vi "mltcoreimaqdx_final.vi"() -> ()   [LabVIEW 2014]
doc: "The Grab VI acquires images continuously and displays the images in an image control using low-level acquisition VIs. A grab is appropriate for high-speed applications in which you need to process only one image at a time."
uses:
  <vilib>/userdefined/High Color/IMAQdx.ctl
  <vilib>/vision/driver/IMAQdx.llb/IMAQdx Acquisition Mode.ctl
  <vilib>/vision/driver/IMAQdx.llb/IMAQdx Buffer Number Mode.ctl
  <vilib>/vision/driver/NI_Vision_Acquisition_Software.lvlib
  <vilib>/vision/NI_Vision_Development_Module.lvlib
panel:
  in  "Add Delay to process loop (ms)":u32
  out "# elements in queue":i32(knob) scale=0.0..250.0
  in  "Range":cluster{"Lower value":sgl, "Upper value":sgl}={"Lower value"=50.0, "Upper value"=140.0} {"Upper value" format="%.2f"; "Lower value" format="%.2f"}
  out "Acquired Image":T1(plugin-control)
  out "Processed Image":T1(plugin-control)
  in  "IMAQdx Session":T2="cam0"
  out "ProcessFrameRate":dbl(knob) scale=0.0..100.0 scale format="%.1f"
  out "ProcessBufferNumber":u32
  out "CameraBuffer Number":u32
  out "CameraFrameRate":dbl(knob) scale=0.0..100.0 scale format="%.1f"
  in  "stop":bool
  # "This example uses NI-IMAQdx to acquire images\nand utilizes a Producer/Consumer loop architecture\nto split the image acquisition and image processing\nbetween multiple threads."
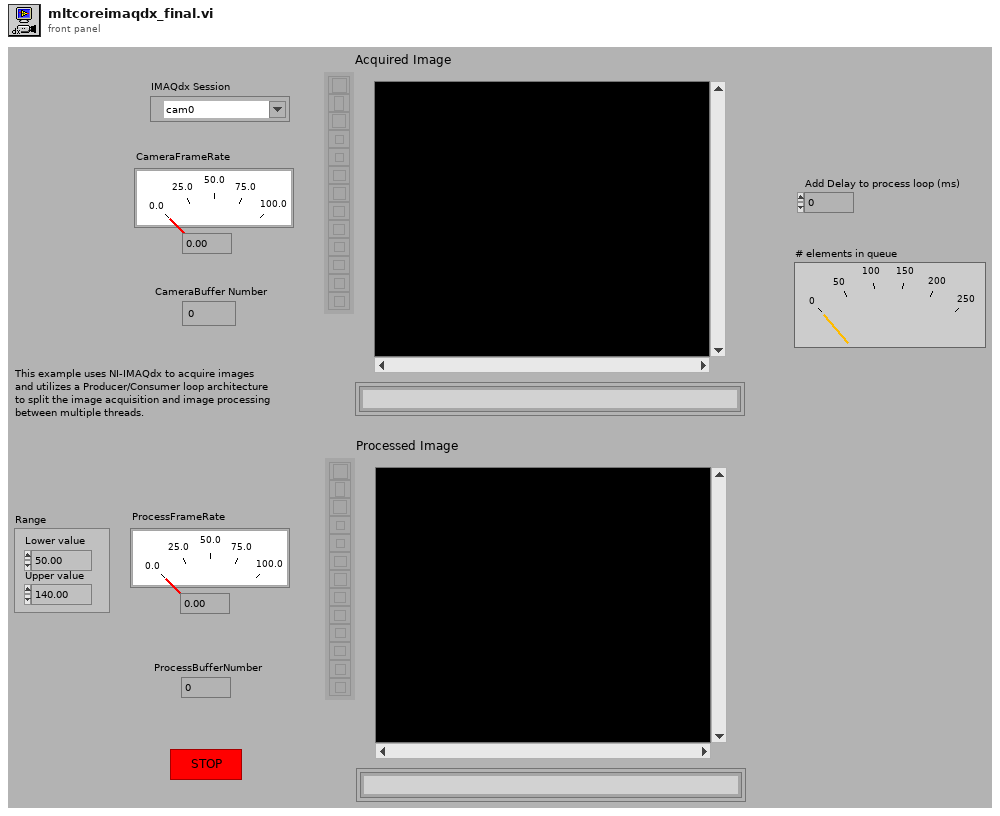
[diagram p1: front panel]
types:
  T1 = typedef "IMAQ Image.ctl" = refnum<image>
  T2 = typedef "IMAQdx.ctl" = refnum<k21>
  T3 = typedef "Image Type" = u32
  T4 = typedef "NI_Vision_Acquisition_Software.lvlib/IMAQdx Acquisition Mode.ctl" = enum32{"One Shot", "Continuous"}
  T5 = typedef "NI_Vision_Acquisition_Software.lvlib/IMAQdx Buffer Number Mode.ctl" = enum32{"Next", "Last", "Buffer Number"}
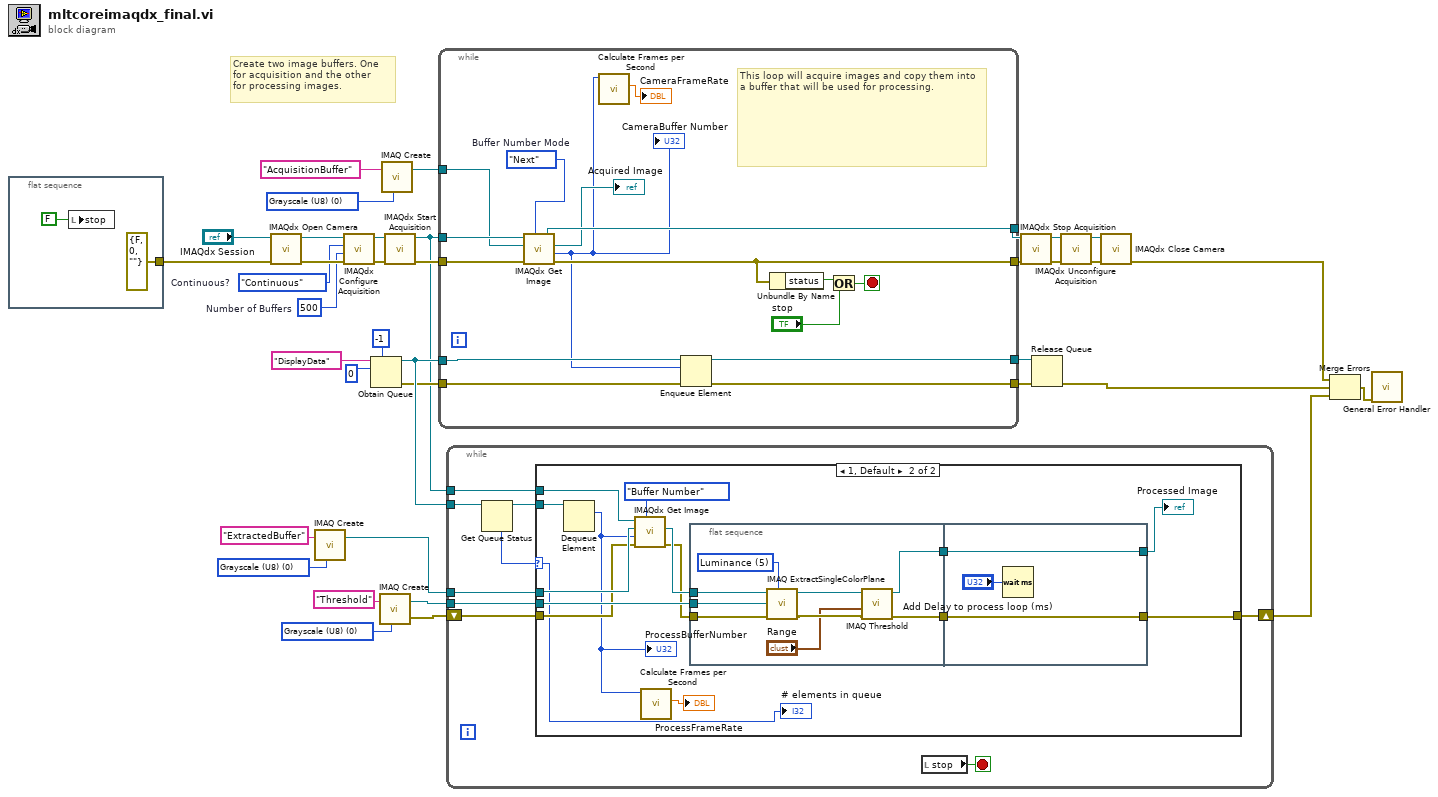
[diagram p0: block diagram]
diagram:
  w4 = T3 0 items=["Grayscale (U8)", "Grayscale (I16)", "Grayscale (SGL)", "Complex (CSG)", "RGB (U32)", "HSL (U32)", "RGB (U64)"] ("Image Type")
  w6 = T3 0 items=["Grayscale (U8)", "Grayscale (I16)", "Grayscale (SGL)", "Complex (CSG)", "RGB (U32)", "HSL (U32)", "RGB (U64)"] ("Image Type")
  w20 = T3 0 items=["Grayscale (U8)", "Grayscale (I16)", "Grayscale (SGL)", "Complex (CSG)", "RGB (U32)", "HSL (U32)", "RGB (U64)"] ("Image Type")
  w34 = u32 500  # Number of Buffers
  w12 = IMAQdx_Acquisition_Mode."Continuous"  # Continuous?
  # "Create two image buffers. One\nfor acquisition and the other\nfor processing images."
  n1 = flat-sequence {
    tunnel: [errorcluster {"status"=FALSE, "code"=0, "source"=""} ("error in")] -> w5
    frame #0 {
      n2 = local write "stop"(FALSE ("stop")) -> ()
    }
  }
  n3 = call <vilib>:"IMAQdx Open Camera.vi"("error in"=w5, "Session In"="IMAQdx Session") -> ("error out"=w35:errorcluster, "Session Out"=w36:T2)  [unwired: 8 in]
  n4 = call "IMAQ Create"("Image Name"="ExtractedBuffer", "Image Type"=w4) -> ("New Image"=w2:T1)  [unwired: 3 in, 1 out]
  n5 = call <vilib>:"IMAQdx Configure Acquisition.vi"("error in"=w35, "Number of Buffers"=w34, "Continuous?"=w12, "Session In"=w36) -> ("error out"=w15:errorcluster, "Session Out"=w11:T2)  [unwired: 6 in]
  n6 = Obtain Queue(max queue size (-1, unlimited)=-1, name (unnamed)="DisplayData", element data type=u32 0) -> (queue out=w23:refnum<queue>, error out=w21:errorcluster)  [unwired: 2 in, 1 out]
  n7 = call "IMAQ Create"("Image Name"="Threshold", "Image Type"=w6) -> ("New Image"=w8:T1, "error out"=w9:errorcluster)  [unwired: 3 in]
  n8 = call "IMAQ Create"("Image Name"="AcquisitionBuffer", "Image Type"=w20) -> ("New Image"=w37:T1)  [unwired: 3 in, 1 out]
  n9 = call <vilib>:"IMAQdx Start Acquisition.vi"("error in"=w15, "Session In"=w11) -> ("error out"=w14:errorcluster, "Session Out"=w1:T2)  [unwired: 8 in]
  n10 = while {
    tunnel: w14 -> [w51]
    tunnel: w1 -> [w52]
    tunnel: [w42] -> w33
    tunnel: w37 -> [w50]
    tunnel: [w49] -> w28
    tunnel: w23 -> [w48]
    tunnel: [w47] -> w24
    tunnel: [w46] -> w22
    tunnel: w21 -> [w45]
    stop <- w55 stop-if-true
    w44 = IMAQdx_Buffer_Number_Mode."Next"  # Buffer Number Mode
    # "This loop will acquire images and copy them into a buffer that will be used for processing."
    n11 = call <vilib>:"IMAQdx Get Image.vi"("Buffer Number Mode (Next)"=w44, "error in"=w51, "Image In"=w50, "Session In"=w52) -> ("error out"=w42:errorcluster, "Buffer Number Out"=w40:u32, "Image Out"=→"Acquired Image":T1, "Session Out"=w49:T2)  [unwired: 4 in]
    "CameraBuffer Number" <- w40
    n12 = call <vilib>:"Calculate Frames per Second.vi"("Buffer Number"=w40) -> ("Processed Frames/s"=→"CameraFrameRate":dbl)  [unwired: 8 in, 2 out]
    n13 = Enqueue Element(queue=w48, element=w40, error in (no error)=w45) -> (queue out=w47:refnum<queue>, error out=w46:errorcluster)  [unwired: 1 in, 1 out]
    n14 = Unbundle By Name(w42) -> ("status"=w54:bool)
    n15 = Or(x=w54, y="stop") -> (x .or. y?=w55:bool)
  }
  n16 = while {
    tunnel: w23 -> [w63]
    tunnel: w2 -> [w60]
    tunnel: w8 -> [w58]
    shift-right: [w57] -> w7
    shift-left: w9 -> [w59]
    tunnel: w1 -> [w56]
    stop <- w64 stop-if-true
    n17 = Get Queue Status(queue=w63) -> (queue out=w61:refnum<queue>, # elements in queue=w62:i32)  [unwired: 2 in, 6 out]
    n18 = case shown="1, Default" w62 {
      selector: w62 -> [_ w70]
      tunnel: w61 -> [_ w80]
      tunnel: w60 -> [_ w74]
      tunnel: w59 -> [w65 w72]
      tunnel: w58 -> [_ w79]
      tunnel: [w65 w78] -> w57
      tunnel: w56 -> [_ w76]
      frame 0 {
      }
      frame 1, Default {
        n19 = Dequeue Element(queue=w80) -> (element=w67:u32)  [unwired: 2 in, 3 out]
        "ProcessBufferNumber" <- w67
        n20 = call <vilib>:"IMAQdx Get Image.vi"("Buffer Number Mode (Next)"=IMAQdx_Buffer_Number_Mode."Buffer Number", "error in"=w72, "Buffer Number In"=w67, "Image In"=w74, "Session In"=w76) -> ("error out"=w71:errorcluster, "Image Out"=w73:T1)  [unwired: 3 in, 2 out]
        n21 = call <vilib>:"Calculate Frames per Second.vi"("Buffer Number"=w67) -> ("Processed Frames/s"=→"ProcessFrameRate":dbl)  [unwired: 8 in, 2 out]
        n22 = flat-sequence {
          tunnel: w79 -> [w89]
          tunnel: w73 -> [w82]
          tunnel: w71 -> [w81]
          tunnel: [w86] -> w69
          tunnel: [w84] -> w68
          tunnel: [w91] -> w77
          tunnel: [w92] -> w78
          tunnel: w69 -> [w92]
          tunnel: w68 -> [w91]
          frame #0 {
            w88 = 5 items=["Red", "Green", "Blue", "Hue", "Saturation", "Luminance", "Value", "Intensity"] ("Color Plane")
            n23 = call "IMAQ ExtractSingleColorPlane"("Color Plane"=w88, "error in (no error)"=w81, "Image Dst"=w89, "Image Src"=w82) -> ("error out"=w87:errorcluster, "Image Dst Out"=w85:T1)  [unwired: 6 in]
            n24 = call "IMAQ Threshold"("error in (no error)"=w87, "Range"="Range", "Image Src"=w85) -> ("error out"=w86:errorcluster, "Image Dst Out"=w84:T1)  [unwired: 7 in]
          }
          frame #1 {
            n25 = Wait (ms)(milliseconds to wait="Add Delay to process loop (ms)") -> ()  [unwired: 1 out]
          }
        }
        "Processed Image" <- w77
        "# elements in queue" <- w70
      }
    }
    n26 = local read "stop"() -> (w64:bool)
  }
  n27 = call <vilib>:"IMAQdx Stop Acquisition.vi"("error in"=w33, "Session In"=w28) -> ("error out"=w29:errorcluster, "Session Out"=w30:T2)  [unwired: 8 in]
  n28 = Release Queue(queue=w24, error in (no error)=w22) -> (error out=w19:errorcluster)  [unwired: 1 in, 2 out]
  n29 = call <vilib>:"IMAQdx Unconfigure Acquisition.vi"("error in"=w29, "Session In"=w30) -> ("error out"=w32:errorcluster, "Session Out"=w31:T2)  [unwired: 8 in]
  n30 = call <vilib>:"IMAQdx Close Camera.vi"("error in"=w32, "Session In"=w31) -> ("error out"=w18:errorcluster)  [unwired: 9 in]
  n31 = Merge Errors(w18, w19, w7) -> (w17:errorcluster)
  n32 = call <vilib>:"General Error Handler.vi"("error in (no error)"=w17) -> ()  [unwired: 10 in, 5 out]
